vi "Motor(SubVI).vi"(6 "Stop":bool, 7 "AI1 and AI2 Channels":u8[](array[numeric]), 8 "error in (no error)":errorcluster, 9 "Duty Cycle (-100 to +100)":dbl(slide) scale=-100.0..100.0, 10 "PWM Channel":u8, 11 "LINX  Input Resource":T1) -> (0 "error out":errorcluster, 2 "Stop output":bool, 3 "LINX Output Resource":T1)   [LabVIEW 2020]
uses:
  <vilib>/MakerHub/LINX/Private/Type Defs/LINX Ref.ctl
  <vilib>/MakerHub/LINX/Private/Type Defs/Platform.ctl
  <vilib>/MakerHub/LINX/Private/Type Defs/Interface.ctl
  <vilib>/MakerHub/LINX/Private/Device/Type Defs/LINX Device Config.ctl
  <vilib>/MakerHub/LINX/Private/Device/Type Defs/TCP Config.ctl
  <vilib>/MakerHub/LINX/Private/Device/Type Defs/Channels.ctl
  <vilib>/MakerHub/LINX/Public/Peripherals/Digital/Digital Write N Chans.vi
  <vilib>/MakerHub/LINX/Public/Peripherals/PWM/PWM Set Duty Cycle 1 Chan.vi
  <vilib>/MakerHub/LINX/Private/Local IO/LinxDigitalWrite.vi
  <vilib>/MakerHub/LINX/Public/Utilities/Check Channel.vi
  <vilib>/MakerHub/LINX/Private/Utilties/Generate Error.vi
  <vilib>/MakerHub/LINX/Public/Peripherals/PWM/PWM Set Duty Cycle N Chans.vi
  <vilib>/MakerHub/LINX/LMH-LINX.lvlib
  <vilib>/MakerHub/LINX/Private/Device/Device.lvlib
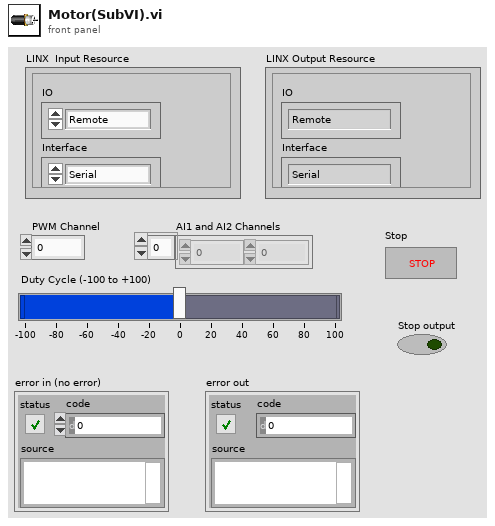
[diagram p1: front panel]
types:
  T1 = typedef "LMH-LINX.lvlib/LINX Ref.ctl" = cluster{"IO":T2, "Interface":T3, "LINX Device Config":T4}
  T2 = typedef "LMH-LINX.lvlib/Platform.ctl" = enum16{"Remote", "Local"}
  T3 = typedef "LMH-LINX.lvlib/Interface.ctl" = enum16{"Serial", "TCP"}
  T4 = typedef "LMH-LINX.lvlib/Device.lvlib/LINX Device Config.ctl" = cluster{"Interface":T3, "COM Port":refnum<visa-resource-name>, "TCP Configuration":T5, "Device Family":u8, "Device ID":u8, "Device Name":string, "TCP Ref":refnum<k5>, "Channels":T6}
  T5 = typedef "LMH-LINX.lvlib/Device.lvlib/TCP Config.ctl" = cluster{"IP Address":string, "Port":u16}
  T6 = typedef "LMH-LINX.lvlib/Channels.ctl" = cluster{"DI":u8[], "DO":u8[], "AI":u8[], "AO":u8[], "PWM":u8[], "QE":u8[], "UART":u8[], "I2C 2":u8[], "SPI":u8[], "CAN":u8[], "Servo":u8[], "AI Ref (V)":dbl, "AI Resolution (Bits)":u8, "AO Ref (V)":dbl, "AO Resolution (Bits)":u8}
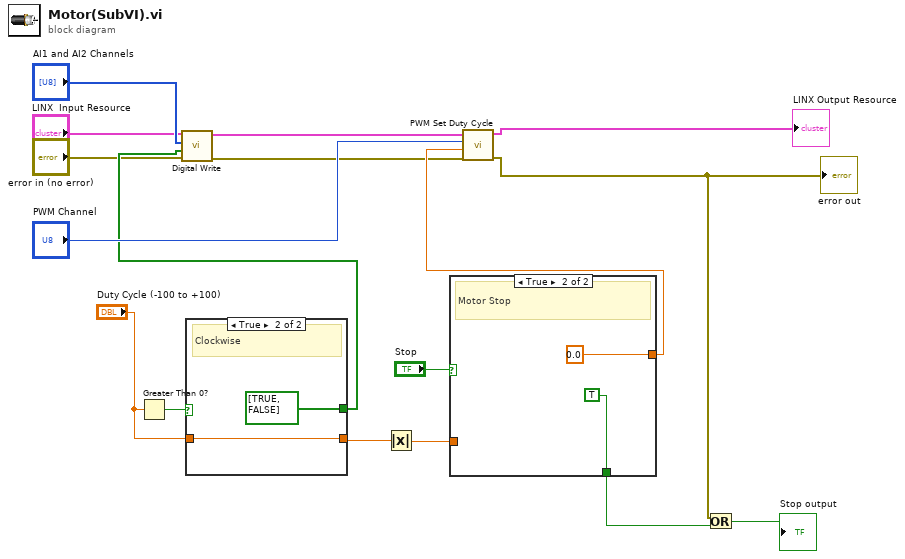
[diagram p0: block diagram]
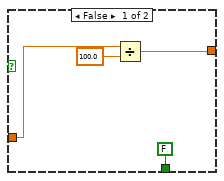
[diagram p2: hidden frame]
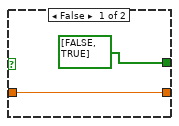
[diagram p3: hidden frame]
diagram:
  n1 = Greater Than 0?(x="Duty Cycle (-100 to +100)") -> (x > 0?=w4:bool)
  n2 = case shown="True" w4 {
    tunnel: [bool[] [FALSE, TRUE] bool[] [TRUE, FALSE]] -> w5
    tunnel: [w18 w20] -> w14
    tunnel: "Duty Cycle (-100 to +100)" -> [w18 w20]
    frame False {
    }
    frame True {
      # "Clockwise"
    }
  }
  n3 = call-poly <vilib>:"Digital Write.vi"("Error In"="error in (no error)", "Values"=w5, "DO Channels"="AI1 and AI2 Channels", "LINX Resource"="LINX  Input Resource") -> ("Error Out"=w9:errorcluster, "LINX Resource"=w8:T1)  [unwired: 6 in]
  n4 = Absolute Value(x=w14) -> (abs(x)=w15:dbl)
  n5 = case shown="True" "Stop" {
    tunnel: w15 -> [w25 _]
    tunnel: [w23 0.0] -> w11
    tunnel: [FALSE TRUE] -> w13
    frame False {
      n6 = Divide(x=w25, y=100.0) -> (x/y=w23:dbl)
    }
    frame True {
      # "Motor Stop"
    }
  }
  n7 = call-poly <vilib>:"PWM Set Duty Cycle.vi"("Error In"=w9, "Duty Cycle (0-1)"=w11, "PWM Channel"="PWM Channel", "LINX Resource"=w8) -> ("Error Out"=w17:errorcluster, "LINX Resource"=→"LINX Output Resource":T1)  [unwired: 6 in]
  "error out" <- w17
  n8 = Or(x=w17, y=w13) -> (x .or. y?=→"Stop output":bool)
